vi "dfd_Group Delay_Gradient Optimization.vi"(6 "modify offset":bool, 7 "parameter":cluster{"epsilon":dbl, "times":i32}={"epsilon"=0.0001, "times"=200}, 8 "error in (no error)":errorcluster, 10 "Coefficients (in)":cluster{"r":dbl[], "theta":dbl[], "offset":dbl}, 11 "Design Info":T1={"p"=2, "freq grid"=[], "d"=[], "weight"=[], "Order"=0, "radius"=1.0}) -> (0 "error out":errorcluster, 1 "Error":dbl, 2 "Coefficients (out)":cluster{"r":dbl[], "theta":dbl[], "offset":dbl})   [LabVIEW 2017, in "NI_DigFilter_Design.lvlib"]
uses:
  <vilib>/addons/Digital Filter Design/NI_DigFilter_Design.lvlib
  <vilib>/addons/Digital Filter Design/_GroupDelay.llb/dfd_Group Delay_Design Info.ctl
  <vilib>/addons/Digital Filter Design/_Misc.llb/dfd_Error Handlers (Single).vi
  <vilib>/addons/Digital Filter Design/_Misc.llb/dfd_X Equal Y (Scalar).vi
  <vilib>/addons/Digital Filter Design/NI_DigFilterLicensed.lvlib
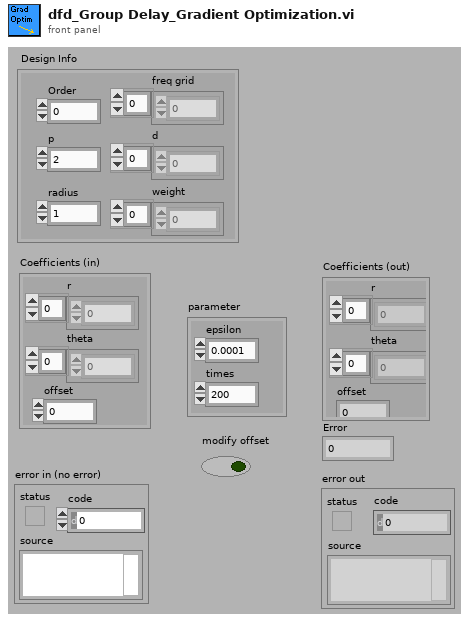
[diagram p1: front panel]
types:
  T1 = typedef "dfd_Group Delay_Design Info.ctl" = cluster{"p":i32, "freq grid":dbl[], "d":dbl[], "weight":dbl[], "Order":i32, "radius":dbl}
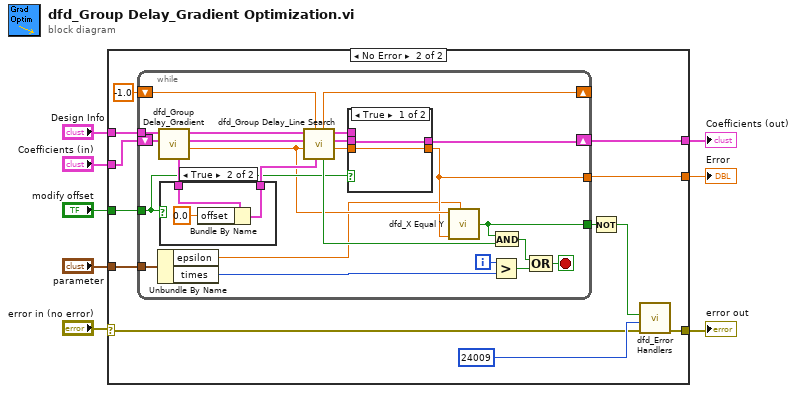
[diagram p0: block diagram]
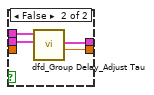
[diagram p3: hidden frame]
diagram:
  n1 = case shown="No Error" "error in (no error)" {
    selector: "error in (no error)" -> [w9 w15]
    tunnel: [_ w20] -> w1
    tunnel: "Design Info" -> [_ w19]
    tunnel: "Coefficients (in)" -> [_ w18]
    tunnel: [_ w17] -> w7
    tunnel: [w9 w14] -> w5
    tunnel: "parameter" -> [_ w11]
    tunnel: "modify offset" -> [_ w10]
    frame Error {
    }
    frame No Error {
      n2 = while {
        shift-right: [w32] -> w20
        shift-left: w18 -> [w45]
        tunnel: w19 -> [w44]
        shift-right: [w28] -> _
        shift-left: -1.0 -> [w29]
        tunnel: [w24] -> w17
        tunnel: [w23] -> w13
        tunnel: w11 -> [w39]
        tunnel: w10 -> [w27]
        i -> [w40]
        stop <- w41 stop-if-true
        n3 = Unbundle By Name(w39) -> ("epsilon"=w22:dbl, "times"=w38:i32)
        n4 = call <vilib>:"dfd_Group Delay_Gradient.vi"("Coefficients"=w45, "Design Info"=w44) -> ("Error"=w25:dbl, "Coefficients (dup)"=w36:cluster{"r":dbl[], "theta":dbl[], "offset":dbl}, "Design Info (dup)"=w37:T1, "Gradients"=w31:cluster{"r":dbl[], "theta":dbl[], "offset":dbl})  [unwired: 6 out]
        n5 = case shown="True" w27 {
          tunnel: w31 -> [w52 w54]
          tunnel: [w52 w53] -> w30
          frame False {
          }
          frame True {
            n6 = Bundle By Name(cluster=w54, "offset"=0.0 ("tau")) -> (w53:cluster{"r":dbl[], "theta":dbl[], "offset":dbl})
          }
        }
        n7 = call <vilib>:"dfd_Group Delay_Line Search.vi"("Gradient"=w30, "steplength (in)"=w29, "error (in)"=w25, "Coefficients (in)"=w36, "Design Info"=w37) -> ("error (out)"=w26:dbl, "Coefficients (out)"=w33:cluster{"r":dbl[], "theta":dbl[], "offset":dbl}, "Design Info (dup)"=w34:T1, "success"=w35:bool, "steplength (out)"=w28:dbl)  [unwired: 2 in]
        n8 = case shown="True" w27 {
          tunnel: w34 -> [_ w51]
          tunnel: w33 -> [w46 w50]
          tunnel: [w46 w49] -> w32
          tunnel: [w47 w48] -> w24
          tunnel: w26 -> [w47 _]
          frame True {
          }
          frame False {
            n9 = call <vilib>:"dfd_Group Delay_Adjust Tau.vi"("Coefficients (in)"=w50, "Design Info"=w51) -> ("Error"=w48:dbl, "Coefficients (out)"=w49:cluster{"r":dbl[], "theta":dbl[], "offset":dbl})  [unwired: 8 out]
          }
        }
        n10 = call-poly <vilib>:"dfd_X Equal Y.vi"("x"=w25, "y"=w24, "esp"=w22) -> ("x = y?"=w23:bool)  [unwired: 4 out]
        n11 = Greater?(x=w40, y=w38) -> (0:w42:bool)
        n12 = And(x=w23, y=w35) -> (x .and. y?=w43:bool)
        n13 = Compound Arithmetic op=OR(w43, w42) -> (w41:bool)
      }
      n14 = Not(x=w13) -> (.not. x?=w12:bool)
      n15 = call-poly <vilib>:"dfd_Error Handlers.vi"("error in (no error)"=w15, "error code"=24009 ("WRN_FAIL_TO_CONVERGE"), "condition failed?"=w12) -> ("error out"=w14:errorcluster)  [unwired: 8 out]
    }
  }
  "Error" <- w7
  "error out" <- w5
  "Coefficients (out)" <- w1
